vi "VeriStand DSF.Transfer Group.Configuration.Create.vi"(8 "error in (no error)":errorcluster, 10 "Section Ref":T1=18446744073709551615 format="%.0x", 11 "Device Ref":T1=18446744073709551615 format="%.0x") -> (0 "error out":errorcluster, 3 "Transfer Group Configuration":refnum<class "VeriStand DSF.Transfer Group.Configuration.lvclass">)   [LabVIEW 2017, in "Data Sharing Framework Engine.lvlib" / "VeriStand DSF.Transfer Group.Configuration.lvclass"]
uses:
  VeriStand DSF.Transfer Group.Configuration.lvclass
  <vilib>/NI Veristand/Custom Device API/Custom Device API.lvlib
  VeriStand DSF.Transfer.Configuration.lvclass
  Builds/Current/Data Sharing Framework Core/Data Sharing Framework Core.lvlibp/Engine/Internal/Configuration Classes/Transfer Group Configuration/Transfer Group Configuration.lvclass
  C:/github/data-sharing-framework/Data Sharing Framework/Builds/Current/Data Sharing Framework Core/Data Sharing Framework Core.lvlibp/Engine/Internal/Configuration Classes/Transfer Configuration/Transfer Configuration.lvclass
  C:/github/data-sharing-framework/Data Sharing Framework/Builds/Current/Data Sharing Framework Core/Data Sharing Framework Core.lvlibp/Engine/Internal/Configuration Classes/Configuration/Configuration.lvclass
  C:/github/data-sharing-framework/Data Sharing Framework/Builds/Current/Data Sharing Framework Core/Data Sharing Framework Core.lvlibp/Engine/Internal/Configuration Classes/Transfer Group Configuration/Transfer Group Configuration.lvclass
  <vilib>/NI Veristand/Custom Device API/Custom Device Item Ref.ctl
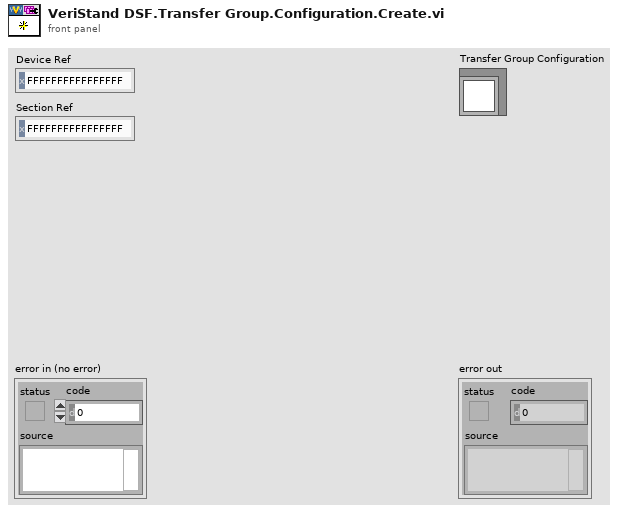
[diagram p1: front panel]
types:
  T1 = typedef "Custom Device API.lvlib/Custom Device Item Ref.ctl" = u64
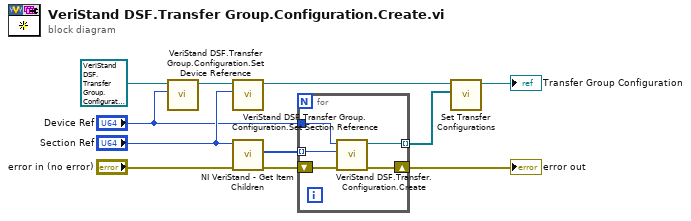
[diagram p0: block diagram]
diagram:
  n1 = call "VeriStand DSF.Transfer Group.Configuration.Set Device Reference.vi"("Device Reference"="Device Ref", "VeriStand DSF.Transfer Group.Configuration in"=refnum<class "VeriStand DSF.Transfer Group.Configuration.lvclass"> refnum ("VeriStand DSF.Plugin.Configuration in")) -> ("VeriStand DSF.Transfer Group.Configuration in"=w3:refnum<class "VeriStand DSF.Transfer Group.Configuration.lvclass">)  [unwired: 9 in]
  n2 = call "VeriStand DSF.Transfer Group.Configuration.Set Section Reference.vi"("Section Ref"="Section Ref", "VeriStand DSF.Transfer Group.Configuration in"=w3) -> ("VeriStand DSF.Transfer Group.Configuration out"=w9:refnum<class "VeriStand DSF.Transfer Group.Configuration.lvclass">)  [unwired: 9 in]
  n3 = call <vilib>:"NI VeriStand - Get Item Children.vi"("error in (no error)"="error in (no error)", "Item Ref in"="Section Ref") -> ("error out"=w10:errorcluster, "Child Refs"=w5:T1[])  [unwired: 6 in, 2 out]
  n4 = for {
    tunnel: w5 -> [w13] mode=indexing
    tunnel: [w15] -> w8 mode=indexing
    shift-right: [w14] -> w6
    shift-left: w10 -> [w16]
    tunnel: "Device Ref" -> [w12]
    n5 = call "VeriStand DSF.Transfer.Configuration.Create.vi"("error in (no error)"=w16, "Section Ref"=w13, "Device Ref"=w12) -> ("error out"=w14:errorcluster, "Transfer Configuration"=w15:refnum<class "VeriStand DSF.Transfer.Configuration.lvclass">)  [unwired: 7 in]
  }
  "error out" <- w6
  n6 = call "Set Transfer Configurations.vi"("Transfer Configurations"=w8, "Transfer Group Configuration in"=w9) -> ("Transfer Group Configuration out"=→"Transfer Group Configuration":refnum<class "VeriStand DSF.Transfer Group.Configuration.lvclass">)  [unwired: 9 in]
